vi "DetectorInitialize.vi"(8 "error in (no error)":errorcluster, 11 "Microscope in":refnum<class "Microscope.lvclass">) -> (0 "error out":errorcluster, 2 "Actual read rate":dbl, 3 "Microscope out":refnum<class "Microscope.lvclass">, 4 "Detector Timebase divisor":i32)   [LabVIEW 2012, in "Microscope.lvclass"]
uses:
  classes/Microscope.lvclass
  classes/Microscope.lvclass/Microscope.ctl
  variables/GlobalUI.vi
  <vilib>/DAQmx/create/channels.llb/DAQmx Create Channel (AI-Voltage-Basic).vi
  <vilib>/DAQmx/configure/timing.llb/DAQmx Timing (Sample Clock).vi
  <resource>/objmgr/daqmx.rc
panel:
  out "Detector read rate":dbl
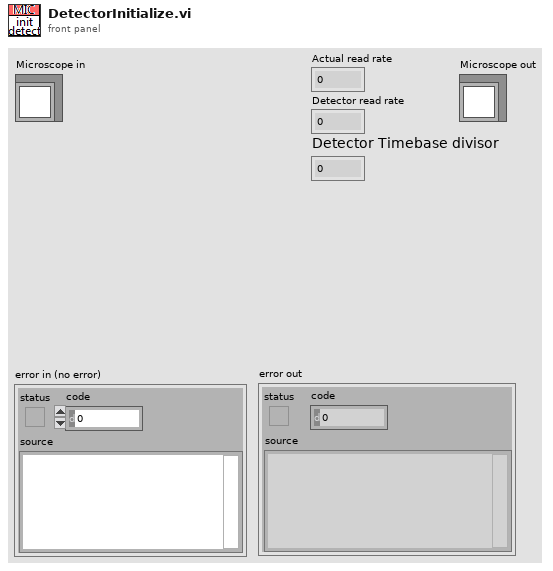
[diagram p1: front panel]
types:
  T1 = typedef "DetectorType.ctl" = enum16{"PMT", "SpectraWiz"}
  T2 = typedef "SyncAlgo.ctl" = cluster{"Pixels/sec":dbl, "Pixel Dwell Time (us)":dbl, "Fill Factor":dbl, "Flyback Pixels":dbl, "Lines/sec":dbl, "Galvo Write rate":dbl, "Galvo Timebase divisor":i32, "total pixels per line":dbl, "Samples to Average":dbl, "Trash Samples":dbl, "Actual samples to Read per Line":dbl, "Detector Read rate":dbl, "Detector Timebase divisor":i32}
  T3 = typedef "HWsettings.ctl" = cluster{"Galvo Channels":tag, "Detector Channels":tag, "Galvo Trigger":tag, "Shutter Lines":tag[], "Max Acquisition Rate":dbl, "Recommended Acquisition Rate":dbl, "Galvo Write Rate":dbl, "Max Timebase Frequency (Hz)":dbl, "MCC Shutter Lines":refnum<k21>[], "Detector Task":refnum<k21>, "Shutter Tasks":refnum<k21>[], "Galvo Task":refnum<k21>, "Digital Image Multiplier":dbl[]}
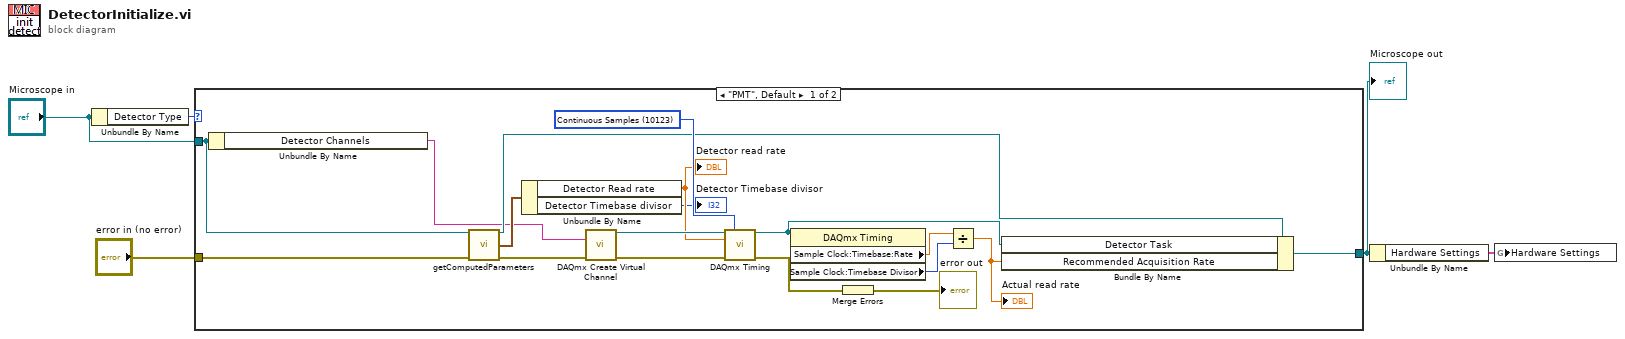
[diagram p0: block diagram]
diagram:
  n1 = Unbundle By Name("Microscope in") -> ("Detector Type"=w1:T1)
  n2 = case shown="\"PMT\", Default" w1 {
    tunnel: "Microscope in" -> [w22 w24]
    tunnel: [w21 w24] -> w5
    tunnel: "error in (no error)" -> [w7 _]
    frame "PMT", Default {
      w20 = 10123 items=["Finite Samples"=10178, "Continuous Samples"=10123, "Hardware Timed Single Point"=12522] ("sample mode")
      n3 = Unbundle By Name(w22) -> ("Detector Channels"=w6:tag)
      n4 = call "getComputedParameters.vi"("Microscope in"=w22, "error in (no error)"=w7) -> ("Microscope out"=w19:refnum<class "Microscope.lvclass">, "Computed Parameters"=w10:T2, "error out"=w17:errorcluster)  [unwired: 10 in, 1 out]
      n5 = Unbundle By Name(w10) -> ("Detector Read rate"=w9:dbl, "Detector Timebase divisor"=→"Detector Timebase divisor":i32)
      "Detector read rate" <- w9
      n6 = call-poly <vilib>:"DAQmx Create Virtual Channel.vi"("physical channels"=w6, "error in"=w17) -> ("task out"=w13:refnum<k21>, "error out"=w18:errorcluster)  [unwired: 12 in]
      n7 = call-poly <vilib>:"DAQmx Timing.vi"("task/channels in"=w13, "sample mode"=w20, "rate"=w9, "error in"=w18) -> ("task out"=w12:refnum<k21>, "error out"=w16:errorcluster)  [unwired: 10 in]
      n8 = property class="DAQmx Timing"(reference=w12) -> ("Sample Clock:Timebase:Rate"=w15:dbl, "Sample Clock:Timebase Divisor"=w14:u32)  [unwired: 1 in, 2 out]
      n9 = Merge Errors(w16) -> (→"error out":errorcluster)
      n10 = Divide(x=w15, y=w14) -> (x/y=w11:dbl)
      "Actual read rate" <- w11
      n11 = Bundle By Name(cluster=w19, "Detector Task"=w12, "Recommended Acquisition Rate"=w11) -> (w21:refnum<class "Microscope.lvclass">)
    }
    frame "SpectraWiz" {
    }
  }
  "Microscope out" <- w5
  n12 = Unbundle By Name(w5) -> ("Hardware Settings"=w4:T3)
  n13 = global write "GlobalUI.vi" "Hardware Settings"(w4) -> ()
